vi "周期设置_总磷总氮.vi"() -> ()   [LabVIEW 2016, in "斯坦道总磷总氮.lvlib"]
uses:
  <vilib>/Utility/miscctls.llb/LVPointTypeDef.ctl
  <vilib>/ptbypt/NI_PtbyPt.lvlib
panel:
  in  "运行周期":T1={"运行模式"=enum."维护模式", "质控频次"=enum."关闭", "空白核查时间"=2, "跨度核查时间"=6, "测量间隔"=240} {"跨度核查时间" items=["00H", "01H", "02H", "03H", "04H", "05H", "06H", "07H", "08H", "09H", "10H", "11H", "12H", "13H", "14H", "15H", "16H", "17H", "18H", "19H", "20H", "21H", "22H", "23H", "关闭"]; "空白核查时间" items=["00H", "01H", "02H", "03H", "04H", "05H", "06H", "07H", "08H", "09H", "10H", "11H", "12H", "13H", "14H", "15H", "16H", "17H", "18H", "19H", "20H", "21H", "22H", "23H", "关闭"]}
  # "运行模式："
  # "质控频次："
  # "零点核查时间："
  # "跨度核查时间："
  # "测量间隔："
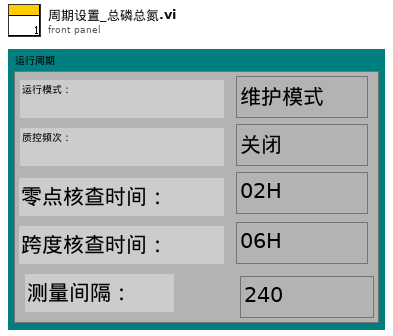
[diagram p1: front panel]
types:
  T1 = cluster{"运行模式":enum16{"维护模式", "常规模式", "应急模式", "质控模式"}, "质控频次":enum16{"关闭", "每天", "星期一", "星期二", "星期三", "星期四", "星期五", "星期六", "星期日"}, "空白核查时间":u16, "跨度核查时间":u16, "测量间隔":u16}
  T2 = typedef "LVPointTypeDef.ctl" = cluster{"Horizontal":i16, "Vertical":i16}
  T3 = enum16{"启动测量", "标样核查", "零点核查", "跨度核查", "空白测试", "平行样测试", "加标回收", "空白校准", "标样校准", "初始化（清洗）", "停止测试", "仪器重启", "校时", "模式设置", "测量间隔设置"}
  T4 = cluster{"系统时间":timestamp, "工作状态":u16, "测量模式":enum16{"待机", "连续模式", "周期模式", "定点模式", "受控模式", "手动模式"}, "告警代码":u16, "故障代码":u16, "日志代码":u16, "软件版本":u16, "F0":sgl, "F1":sgl, "F2":sgl, "F3":sgl, "T":sgl, "H":sgl, "id":u16, "flowid":u16, "量程":u16, "总磷控温温度1":sgl, "营养盐控温温度2":sgl, "ADC":sgl}
  T5 = enum16{"关闭", "每天", "星期一", "星期二", "星期三", "星期四", "星期五", "星期六", "星期日"}
  T6 = typedef "LVDateTimeRec.ctl" = cluster{"秒数的小数部分":dbl, "秒":i32, "分":i32, "时":i32, "日":i32, "月":i32, "年":i32, "天数（周）":i32, "天数（年）":i32, "DST":i32}
  T7 = cluster{"运行模式":enum16{"维护模式", "常规模式", "应急模式", "质控模式", "性能测试"}, "质控频次":enum16{"关闭", "每天", "星期一", "星期二", "星期三", "星期四", "星期五", "星期六", "星期日"}, "空白核查时间":u16, "跨度核查时间":u16, "测量间隔":u16}
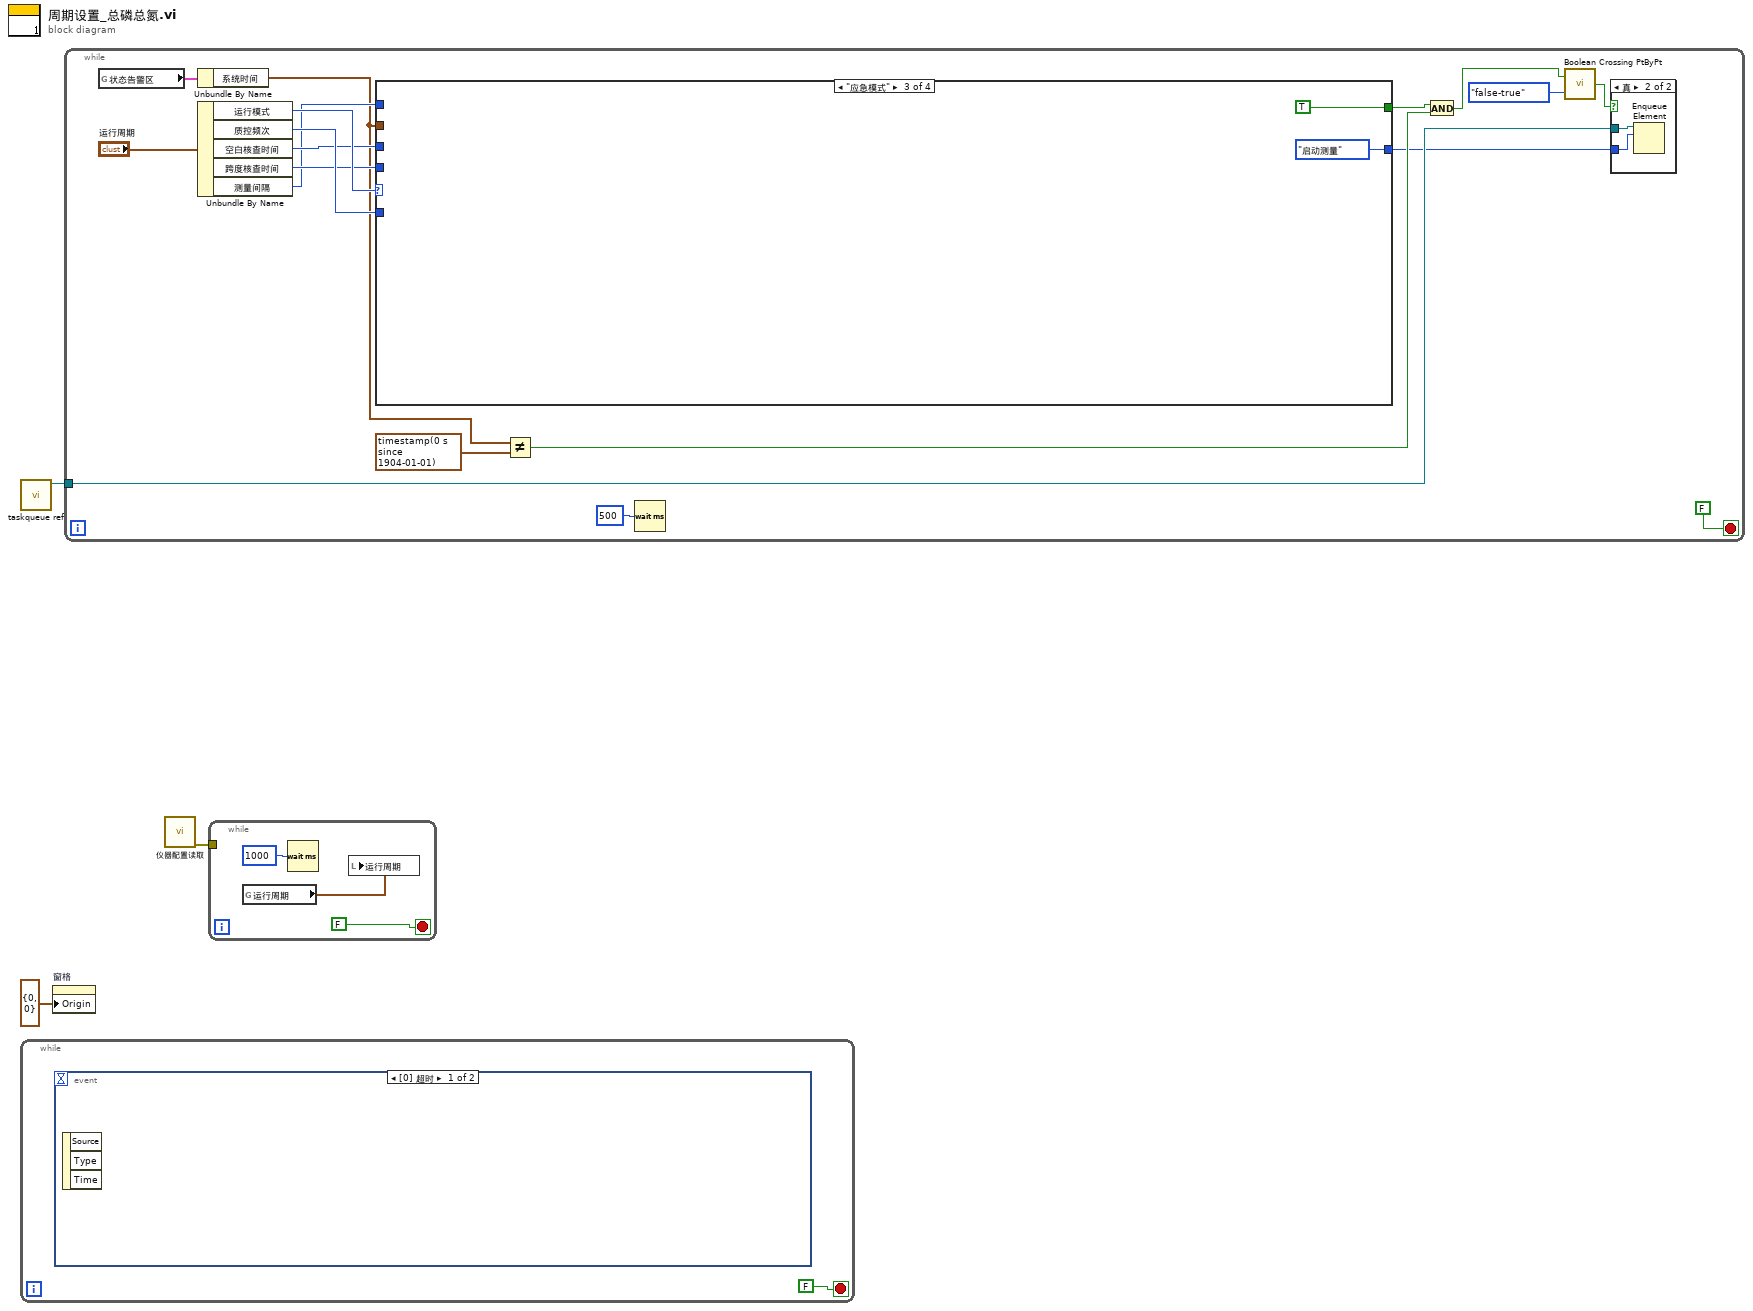
[diagram p0: block diagram]
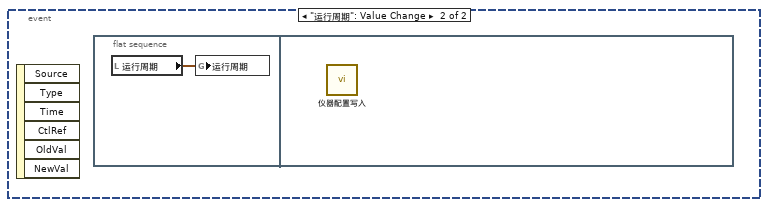
[diagram p2: hidden frame]
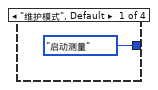
[diagram p4: hidden frame]
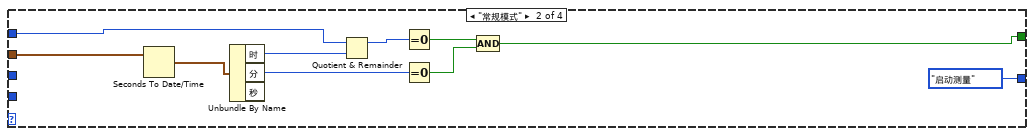
[diagram p5: hidden frame]
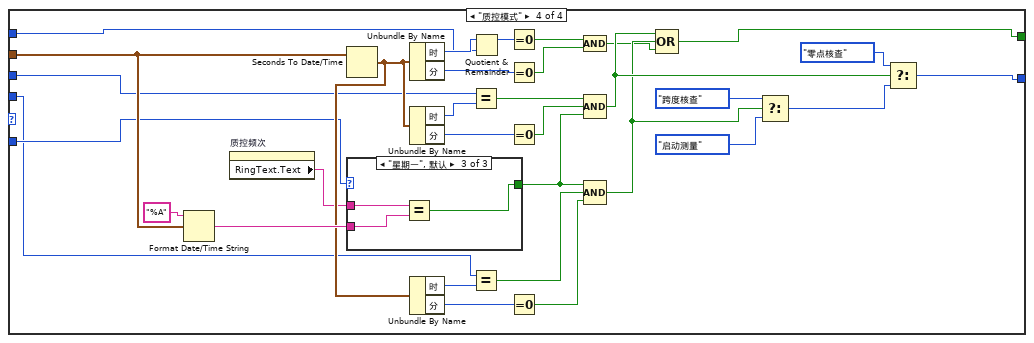
[diagram p6: hidden frame]
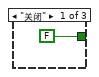
[diagram p7: hidden frame]
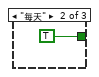
[diagram p8: hidden frame]
diagram:
  n1 = call "taskqueue ref.vi"() -> ("队列输出"=w1:refnum<queue>)  [unwired: 10 in, 1 out]
  n2 = while {
    stop <- FALSE stop-if-true
    n3 = event shown="[0] 超时" {
      selector: _ -> [_ _]
      dyn-events: _ -> [_ _]
      timeout: _ -> [_ _]
      event Timeout {
        n4 = event-data() -> ()  [unwired: 1 in, 3 out]
      }
      event "运行周期": Value Change {
        n5 = event-data() -> ()  [unwired: 1 in, 6 out]
        n6 = flat-sequence {
          frame #0 {
            n7 = local read "运行周期"() -> (w5:T1)
            n8 = global write "总磷总氮断电保存全局变量.vi" "运行周期"(w5) -> ()
          }
          frame #1 {
            n9 = call "仪器配置写入.vi"() -> ()  [unwired: 11 in, 1 out]
          }
        }
      }
    }
  }
  n10 = property on="窗格" class="Pane"("Origin"=T2 {"Horizontal"=0, "Vertical"=0} ("原点")) -> ()  [unwired: 2 in, 2 out]
  n11 = while {
    tunnel: w1 -> [w11]
    stop <- FALSE stop-if-true
    n12 = global read "VAR总磷总氮全局变量.vi" "状态告警区"() -> (w15:T4)
    n13 = Unbundle By Name(w15) -> ("系统时间"=w14:timestamp)
    n14 = Unbundle By Name("运行周期") -> ("运行模式"=w21:enum16{"维护模式", "常规模式", "应急模式", "质控模式"}, "质控频次"=w20:T5, "空白核查时间"=w19:u16, "跨度核查时间"=w18:u16, "测量间隔"=w17:u16)
    n15 = case shown="\"应急模式\"" w21 {
      tunnel: w14 -> [_ w36 _ w70]
      tunnel: w17 -> [_ w29 _ w41]
      tunnel: [_ w32 TRUE w56] -> w16
      tunnel: [T3."启动测量" ("控制命令") T3."启动测量" ("控制命令") T3."启动测量" ("控制命令") w52] -> w10
      tunnel: w20 -> [_ _ _ w49]
      tunnel: w19 -> [_ _ _ w48]
      tunnel: w18 -> [_ _ _ w47]
      frame "维护模式", Default {
      }
      frame "常规模式" {
        n16 = Seconds To Date/Time(time stamp (now)=w36) -> (date time rec=w35:T6)  [unwired: 1 in]
        n17 = Unbundle By Name(w35) -> ("时"=w28:i32, "分"=w34:i32)  [unwired: 1 out]
        n18 = Quotient & Remainder(x=w29, y=w28) -> (x-y*floor(x/y)=w30:i32)  [unwired: 1 out]
        n19 = Equal To 0?(x=w30) -> (x = 0?=w27:bool)
        n20 = Equal To 0?(x=w34) -> (x = 0?=w33:bool)
        n21 = Compound Arithmetic op=AND ("复合运算")(w27, w33) -> (w32:bool)
      }
      frame "应急模式" {
      }
      frame "质控模式" {
        n22 = Format Date/Time String(time format string (%c)="%A" ("时间格式字符串(%c)"), seconds (now)=w70) -> (date/time string=w68:string)  [unwired: 1 in]
        n23 = property on="质控频次" class="Enum (严格)"() -> ("RingText.Text"=w43:string)  [unwired: 2 in, 2 out]
        n24 = Seconds To Date/Time(time stamp (now)=w70) -> (date time rec=w59:T6)  [unwired: 1 in]
        n25 = case shown="\"星期一\", 默认" w49 {
          tunnel: w68 -> [_ _ w75]
          tunnel: [FALSE TRUE w74] -> w50
          tunnel: w43 -> [_ _ w73]
          frame "关闭" {
          }
          frame "每天" {
          }
          frame "星期一", Default {
            n26 = Equal?(x=w73, y=w75) -> (x = y?=w74:bool)
          }
        }
        n27 = Unbundle By Name(w59) -> ("时"=w42:i32, "分"=w67:i32)
        n28 = Unbundle By Name(w59) -> ("时"=w65:i32, "分"=w64:i32)
        n29 = Unbundle By Name(w59) -> ("时"=w60:i32, "分"=w61:i32)
        n30 = Equal?(x=w48, y=w65) -> (x = y?=w63:bool)
        n31 = Equal?(x=w47, y=w60) -> (x = y?=w58:bool)
        n32 = Quotient & Remainder(x=w42, y=w41) -> (x-y*floor(x/y)=w40:i32)  [unwired: 1 out]
        n33 = Equal To 0?(x=w40) -> (x = 0?=w39:bool)
        n34 = Equal To 0?(x=w67) -> (x = 0?=w66:bool)
        n35 = Equal To 0?(x=w64) -> (x = 0?=w62:bool)
        n36 = Equal To 0?(x=w61) -> (x = 0?=w57:bool)
        n37 = Compound Arithmetic op=AND ("复合运算")(w39, w66) -> (w51:bool)
        n38 = Compound Arithmetic op=AND ("复合运算")(w63, w62, w50) -> (w55:bool)
        n39 = Compound Arithmetic op=AND ("复合运算")(w50, w58, w57) -> (w54:bool)
        n40 = Compound Arithmetic op=OR ("复合运算")(w55, w54, w51) -> (w56:bool)
        n41 = Select(t=T3."跨度核查" ("控制命令"), s=w54, f=T3."启动测量" ("控制命令")) -> (s? t:f=w53:T3)
        n42 = Select(t=T3."零点核查" ("控制命令"), s=w55, f=w53) -> (s? t:f=w52:T3)
      }
    }
    n43 = Not Equal?(x=w14, y=timestamp(0 s since 1904-01-01)) -> (x != y?=w12:bool)
    n44 = Wait (ms)(milliseconds to wait=u32 500 ("等待时间（毫秒）")) -> ()  [unwired: 1 out]
    n45 = And(x=w16, y=w12) -> (x .and. y?=w9:bool)
    n46 = call <vilib>:"Boolean Crossing PtByPt.vi"("direction"=enum16{"either", "false-true", "true-false"}."false-true", "input"=w9) -> ("crossing"=w8:bool)  [unwired: 1 in]
    n47 = case shown="真" w8 {
      tunnel: w11 -> [_ w25]
      tunnel: w10 -> [_ w24]
      frame False {
      }
      frame True {
        n48 = Enqueue Element(queue=w25, element=w24) -> ()  [unwired: 2 in, 3 out]
      }
    }
  }
  n49 = call "仪器配置读取.vi"() -> ("error out"=w2:errorcluster)  [unwired: 11 in]
  n50 = while {
    tunnel: w2 -> [_]
    stop <- FALSE stop-if-true
    n51 = global read "总磷总氮断电保存全局变量.vi" "运行周期"() -> (w76:T7)
    n52 = Wait (ms)(milliseconds to wait=u32 1000 ("等待时间（毫秒）")) -> ()  [unwired: 1 out]
    n53 = local write "运行周期"(w76) -> ()
  }
